vi "Write Async Call Method.vi"(8 "error in (no error)":errorcluster, 10 "Async Method":T1, 11 "Async Message Msg in":refnum<class "Async Message.lvclass">) -> (0 "error out":errorcluster, 3 "Async Message Msg out":refnum<class "Async Message.lvclass">)   [LabVIEW 2023, in "Async Methods Actor.lvlib" / "Async Message.lvclass"]
doc: "This property enumeration can take values \"Call and Collect\" and \"Call and Forget\". In the former case the \"Async Methods Actor\" will track execution of the methods by waiting for their completion, in the latter case instead the actor will not wait for their completion but will just count their launch."
uses:
  Async Message.lvclass
  Async Methods Actor/Async Call Method.ctl
  Async Message.lvclass/Async Message.ctl
  Async Methods Actor/Async Methods Actor.lvclass
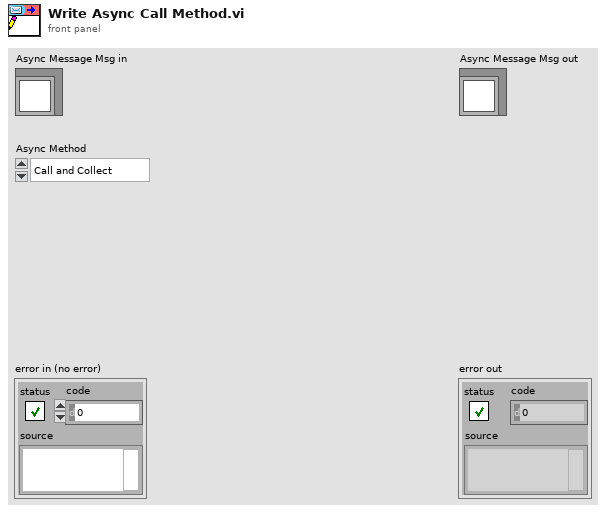
[diagram p1: front panel]
types:
  T1 = typedef "Async Methods Actor.lvlib/Async Methods Actor.lvclass/Async Call Method.ctl" = enum16{"Call and Collect", "Call and Forget"}
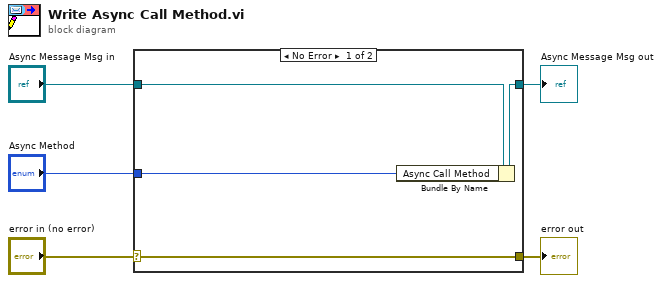
[diagram p0: block diagram]
diagram:
  n1 = case shown="No Error" "error in (no error)" {
    selector: "error in (no error)" -> [w9 w10]
    tunnel: [w9 w10] -> w4
    tunnel: [w7 w11] -> w2
    tunnel: "Async Message Msg in" -> [w8 w11]
    tunnel: "Async Method" -> [w6 _]
    frame No Error {
      n2 = Bundle By Name(cluster=w8, "Async Call Method"=w6) -> (w7:refnum<class "Async Message.lvclass">)
    }
    frame Error {
    }
  }
  "error out" <- w4
  "Async Message Msg out" <- w2
